vi "Pitch Shifting in Real Time.vi"(8 "Pitch multiplier":dbl(slide)=1.0 min=0.5 max=2.0 step=0.01 scale=0.5..2.0, 9 "output waveform 2":waveform(dbl)) -> (1 "Pitch Shifted Speech":dbl[](graph), 2 "Original Speech":dbl[](graph), 3 "output waveform":waveform(dbl))   [LabVIEW 2024]
doc: "This example shows how to configure a sound card device, continuously acquire and play sound data, and shift the pitch of a normal speech with the TFA Online Gabor Transform VI and Online Gabor Expansion VI.\n\n<b>Instructions:</b>\n1) Run this VI.\n2) Adjust the <b>Pitch multiplier</b>.\n3) Speak into the microphone.\n4) Listen to the output pitch shifted speech.\n5) Browse the Block Diagram of this example to learn how to use the TFA Online Gabor Transform VI and TFA Online Gabor Expansion VI."
uses:
  <vilib>/addons/Time Frequency Analysis/Transform.llb/TFA Online Gabor Transform (Real).vi
  <vilib>/addons/Time Frequency Analysis/Transform.llb/TFA Online Gabor Expansion (Real).vi
  <vilib>/Analysis/2dsp.llb/Resample (constant to constant,single -channel).vi
  <vilib>/addons/Time Frequency Analysis/Spectrogram.llb/TFA Online STFT Spectrogram (Waveform).vi
  <vilib>/addons/_Advanced Signal Processing/NI_AdvSigProcTFA.lvlib
  <vilib>/Analysis/NI_AALPro.lvlib
panel:
  out "aspt-left-top":bool
  # "*** This example requires sound card, microphone and headset installed in your computer ***\n Select Help>>Show Context Help and move the cursor over the VI icon of this example for more information."
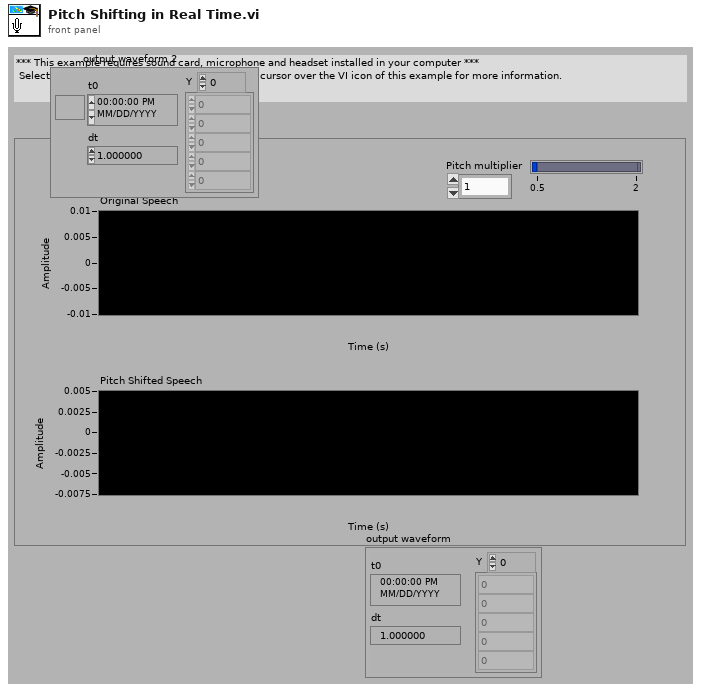
[diagram p1: front panel]
types:
  T1 = cluster{"synthesis window":dbl[], "dM (time steps)":i32, "N (frequency bins)":i32}
  T2 = cluster{"analysis window":dbl[], "dM (time steps)":i32, "N (frequency bins)":i32}
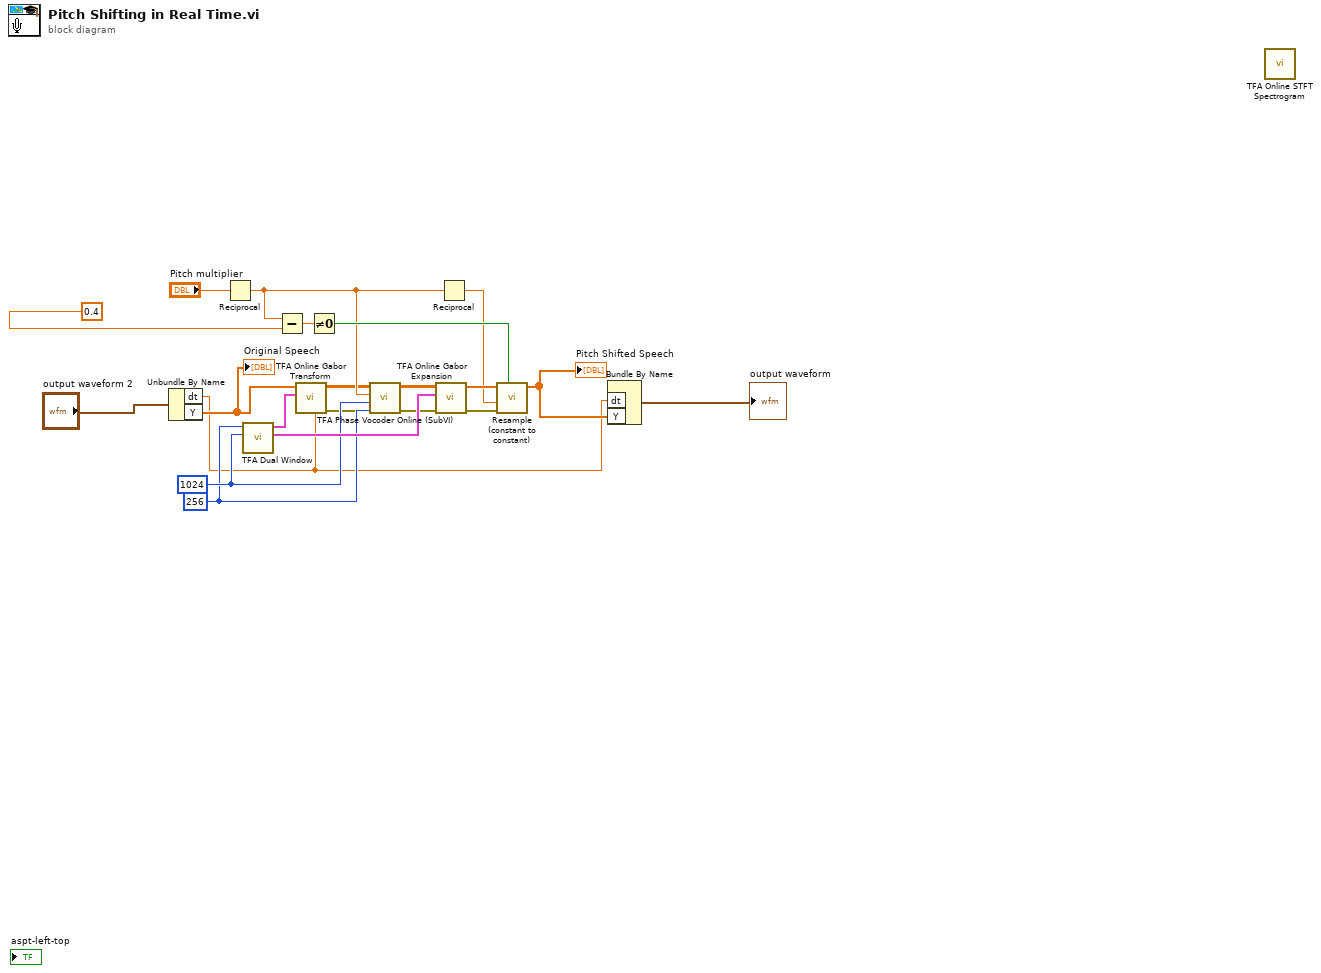
[diagram p0: block diagram]
diagram:
  w10 = 256 ("hop")
  w11 = 1024 ("N")
  n1 = Unbundle By Name("output waveform 2") -> ("dt"=w5:dbl, "Y"=w7:dbl[])
  "Original Speech" <- w7
  n2 = Reciprocal(x="Pitch multiplier") -> (1/x=w17:dbl)
  n3 = call <vilib>:"TFA Dual Window.vi"("N (frequency bins)"=w11, "dM (time steps)"=w10) -> ("synthesis info"=w15:T1, "analysis info"=w16:T2)  [unwired: 2 in, 6 out]
  n4 = Subtract(x=w17, y=0.4) -> (x-y=w20:dbl)
  n5 = call-poly <vilib>:"TFA Online Gabor Transform.vi"("sampling rate"=w5, "transform info"=w16, "signal"=w7) -> ("error out"=w9:errorcluster, "Gabor coef"=w4:cdb[][])  [unwired: 1 in, 6 out]
  n6 = Not Equal To 0?(x=w20) -> (x != 0?=w18:bool)
  n7 = call "TFA Phase Vocoder Online (SubVI).vi"("hop"=w10, "N"=w11, "squeeze"=w17, "STFT coef in"=w4) -> ("STFT coef out"=w14:cdb[][])  [unwired: 7 out]
  n8 = call-poly <vilib>:"TFA Online Gabor Expansion.vi"("error in (no error)"=w9, "expansion info"=w15, "Gabor coef"=w14) -> ("error out"=w8:errorcluster, "signal"=w13:dbl[])  [unwired: 7 out]
  n9 = Reciprocal(x=w17) -> (1/x=w12:dbl)
  n10 = call-poly <vilib>:"Resample (constant to constant).vi"("reset?"=w18, "error in (no error)"=w8, "dt"=w12, "X"=w13) -> ("Y"=w6:dbl[])  [unwired: 3 in, 4 out]
  "Pitch Shifted Speech" <- w6
  n11 = Bundle By Name("dt"=w5, "Y"=w6) -> (→"output waveform":waveform(dbl))  [unwired: 1 in]
  n12 = call-poly <vilib>:"TFA Online STFT Spectrogram.vi"() -> ()  [unwired: 4 in, 8 out]
